vi "Read Sync Group.vi"(8 "error in (no error)":errorcluster, 11 "DriveMotorsRight in":refnum<class "DriveMotorsRight.lvclass">) -> (0 "error out":errorcluster, 2 "Sync Group":u8=128 format="%x", 3 "DriveMotorsRight out":refnum<class "DriveMotorsRight.lvclass">)   [LabVIEW 2013, in "DriveMotorsRight.lvclass"]
uses:
  DriveMotorsRight.lvclass
  DriveMotorsRight.lvclass/DriveMotorsRight.ctl
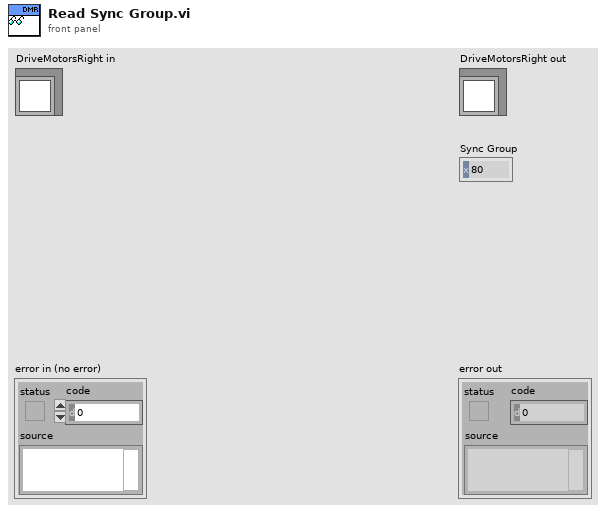
[diagram p1: front panel]
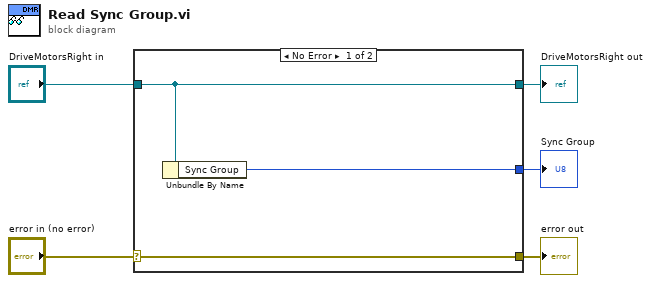
[diagram p0: block diagram]
diagram:
  n1 = case shown="No Error" "error in (no error)" {
    selector: "error in (no error)" -> [w8 w9]
    tunnel: [w8 w9] -> w4
    tunnel: [w7 w10] -> w2
    tunnel: "DriveMotorsRight in" -> [w7 w10]
    tunnel: [w6 _] -> w1
    frame No Error {
      n2 = Unbundle By Name(w7) -> ("Sync Group"=w6:u8)
    }
    frame Error {
    }
  }
  "error out" <- w4
  "DriveMotorsRight out" <- w2
  "Sync Group" <- w1
